vi "FPGA_UtilitiesRead LocalTime.vi"(8 "error in (no error)":errorcluster) -> (0 "error out":errorcluster, 3 "LocalTime":u32)   [LabVIEW 2017]
uses:
  <vilib>/rvi/errors/niLvFpgaAdjustHostInterfaceError.vi
  <vilib>/Utility/error.llb/Error Cluster From Error Code.vi
  <vilib>/Rock Robotics/SystemInterfaces/System/FPGA_SystemFRC FPGA Ref.ctl
  <vilib>/rvi/interface/nirviReadWriteControl/nirviReadWriteControl.xnode
  NiFpgaLv.dll
  <vilib>/rvi/interface/Simulation/niFpgaSimulationCallBeginRW.vi
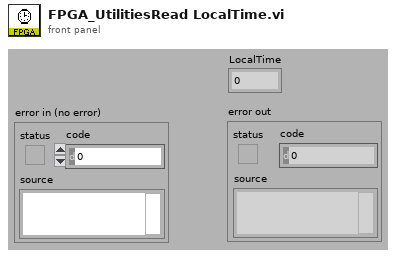
[diagram p1: front panel]
types:
  T1 = typedef "FPGA_SystemFRC FPGA Ref.ctl" = refnum<k20>
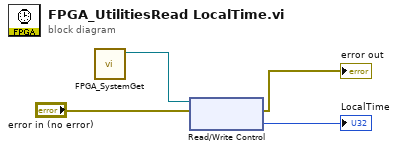
[diagram p0: block diagram]
diagram:
  n1 = call <vilib>:"FPGA_SystemGet.vi"() -> ("FRC FPGA Ref"=w1:T1)  [unwired: 11 in]
  n2 = xnode "Read/Write Control"("FPGA VI Reference In"=w1, "error in"="error in (no error)") -> ("error out"=→"error out":errorcluster, "LocalTime"=→"LocalTime":u32)  [unwired: 1 out]
